vi "ParseArguments.vi"(8 "error in (no error)":errorcluster, 10 "CliArguments":string[](array[string]), 11 "ArgumentParser in":refnum<class "ArgumentParser.lvclass">) -> (0 "error out":errorcluster, 2 "ParsedData":refnum<class "ParsedData.lvclass">, 3 "ArgumentParser out":refnum<class "ArgumentParser.lvclass">)   [LabVIEW 2022 SP3, in "ArgumentParser.lvlib" / "ArgumentParser.lvclass"]
uses:
  ArgumentParser.lvclass
  C:/Users/jakub/repos/gh/sw4sys/lv-argument-parser/PythonWrapper/Source/PythonSession/PythonSession.lvclass
  C:/Users/jakub/repos/gh/sw4sys/lv-argument-parser/PythonWrapper/Source/PythonWrapper/PythonWrapper.lvclass
  C:/Users/jakub/repos/gh/sw4sys/lv-argument-parser/ArgumentParser/Source/ArgparseWrapper/ArgparseWrapper.lvclass
  PythonWrapper/Source/PythonSession/PythonSession.lvclass/PythonSession.ctl
  PythonWrapper/Source/PythonWrapper/PythonWrapper.lvclass/PythonWrapper.ctl
  ArgparseWrapper/ArgparseWrapper.lvclass/ArgparseWrapper.ctl
  ArgumentParser.lvclass/ArgumentParser.ctl
  PythonWrapper/Source/PythonSession/Read PythonSession.vi
  PythonWrapper/Source/PythonWrapper/Read ModulePath.vi
  ArgparseWrapper/Read FunctionParseArgs.vi
  Read Name.vi
  ParsedData/ParsedData.lvclass
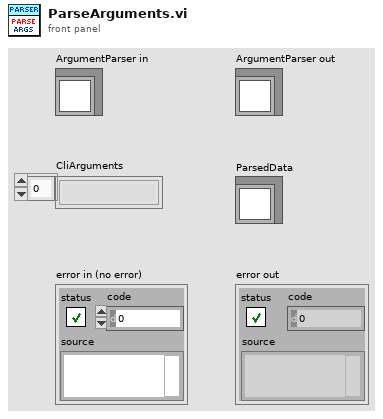
[diagram p1: front panel]
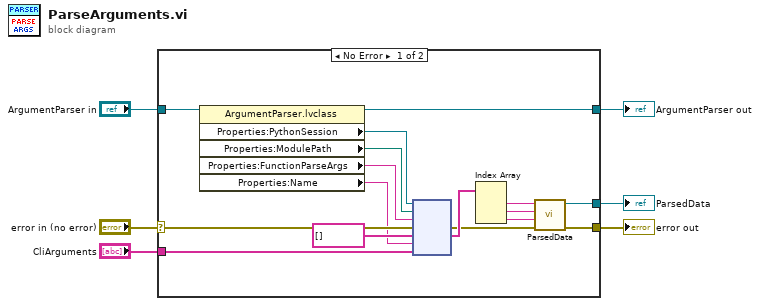
[diagram p0: block diagram]
diagram:
  n1 = case shown="No Error" "error in (no error)" {
    selector: "error in (no error)" -> [w22 w24]
    tunnel: [w7 w24] -> w5
    tunnel: [w17 w23] -> w3
    tunnel: "ArgumentParser in" -> [w21 w23]
    tunnel: "CliArguments" -> [w19 _]
    tunnel: [w9 _] -> w1
    frame No Error {
      n2 = property class="ArgumentParser.lvclass"(reference=w21) -> (reference out=w17:refnum<class "ArgumentParser.lvclass">, "Properties:PythonSession"=w15:refnum<k35>, "Properties:ModulePath"=w13:path, "Properties:FunctionParseArgs"=w14:string, "Properties:Name"=w16:string)  [unwired: 1 in, 1 out]
      n3 = node(w15, w13, w14, w22, string[] [], w16, w19) -> (w8:errorcluster, w18:string[])  [unwired: 2 in, 3 out]
      n4 = Index Array(array=w18) -> (element #1=w12:string, element #2=w10:string, element #3=w11:string)  [unwired: 3 in]
      n5 = call "ParsedData.vi"("error in (no error)"=w8, "StdErr"=w11, "StdOut"=w10, "Arguments"=w12) -> ("error out"=w7:errorcluster, "ParsedData"=w9:refnum<class "ParsedData.lvclass">)  [unwired: 6 in]
    }
    frame Error {
    }
  }
  "error out" <- w5
  "ArgumentParser out" <- w3
  "ParsedData" <- w1
